vi "FPGA SECONDARY 9049.vi"() -> ()   [LabVIEW 2018]
doc: "This FPGA Main VI contains a control loop running in parallel with an RT watchdog loop.\n- The Control Loop performs control calculations on four input channels in parallel, and outputs the results to four output channels.\n- The RT Watchdog Loop checks for a periodic 'pet' from the RT Main VI to ensure communications between RT and FPGA are maintained."
uses:
  <vilib>/LabVIEW Targets/FPGA/cRIO/shared/nicrio_ModuleControls/nicrio_cRIO-9237_DataRatesRing.ctl
  <vilib>/LabVIEW Targets/FPGA/cRIO/shared/nicrio_ModuleControls/nicrio_cRIO-9237_ExcitationVoltageRing.ctl
  <vilib>/rvi/Emulation/niFpgaGetClockAttributes.vi
  <vilib>/rvi/Emulation/niFpgaSctlEmulationGetInTimedLoop.vi
  <vilib>/rvi/Emulation/niFpgaEmulationReportErrorSimple.vi
  <vilib>/rvi/eio/common/nirviEmuTemplatePropertySet_errors.vi
  <vilib>/rvi/interface/RandomDataEmulation/niFpgaRandomDataHandleErrors.vi
  <vilib>/rvi/Emulation/niFpgaProcessEmulError.vi
  <vilib>/rvi/eio/common/nirviEmuTemplateMethod_errors.vi
  <vilib>/rvi/Emulation/niFpgaCriticalErrorInLSC.vi
  <vilib>/rvi/eio/common/nirviEmuTemplatePropertyGet_noerrors.vi
  <vilib>/eio/EIOPropertyNode/EIOPropertyNode.xnode
  <vilib>/rvi/DataTransferAndStorage/Container/XNode/niFpgaContainer.xnode
  <vilib>/rvi/interface/RandomDataEmulation/nirviRandomDataFpgaReadWriteTemplate.vi
  <vilib>/eio/EIONode/EIONode.xnode
  <vilib>/eio/EIOMethodNode/EIOMethodNode.xnode
  <vilib>/rvi/eio/common/nirviEmuTemplatePropertyGet_errors.vi
  <vilib>/rvi/eio/common/nirviEmuTemplatePropertySet_noerrors.vi
  COMET  Extra Programs/FPGA Time Keeper/FPGA Timekeeper.lvlib
panel:
  out "UTC Offset Valid":bool
  out "FPGA time (ns)":u64
  out "PPS Timestamp (TAI)":u64
  out "UTC Offset":i8
  out "Antenna Status":T1(ring)
  out "offset from time reference":i32
  out "FPGA Timekeeper locked":bool
  out "FPGA Error 3":errorcluster
  out "Finished 2":bool
  out "Module Underflow 2":bool
  out "DMA FIFO Full 2":bool
  out "Different Channel Count 2":bool
  out "Actual Loop Period (ticks) 2":u32
  in  "9222 Sample Time":u32=2 caption="Sample Time 9222 [microS]"
  in  "stop":bool
  out "First Read 2":bool
  in  "Number of Channels 9222":i32=29
  out "FPGA Error 2":errorcluster
  in  "Samples per Channel":u32=1000
  in  "Finite?":bool=TRUE
  in  "Shunt Cal Enable":bool
  out "x+y 7":u8
  out "x+y 6":u8
  out "x+y 5":u8
  out "x+y 4":u8
  out "x+y 3":u8
  out "x+y":u8
  out "Preloop":i32
  out "Counter":i32
  out "appended array":fxp<+/-,24,-4>[](array[numeric])
  in  "Excitation Voltage":T2=1 items=["2.5 Volts", "3.3 Volts", "5.0 Volts", "10.0 Volts", "External Excitation"]
  out "FPGA Error":errorcluster
  out "Finished":bool
  in  "Stop":bool
  out "Module Underflow":bool
  out "DMA FIFO Full":bool
  out "Different Channel Count":bool
  out "First Read":bool
  in  "Number of Channels 9237":i32=8
  in  "Data Rate 9237":T3=1 items=["50.000 kS/s (NI 9237)"=1, "25.000 kS/s (NI 9237)"=2, "16.667 kS/s (NI 9237)"=3, "12.500 kS/s (NI 9237)"=4, "10.000 kS/s (NI 9237)"=5, "8.333 kS/s (NI 9237)"=6, "7.143 kS/s (NI 9237)"=7, "6.250 kS/s (NI 9237)"=8, "5.556 kS/s (NI 9237)"=9, "5.000 kS/s (NI 9237)"=10, "4.545 kS/s (NI 9237)"=11, "4.167 kS/s (NI 9237)"=12, "3.846 kS/s (NI 9237)"=13, "3.571 kS/s (NI 9237)"=14, "3.333 kS/s (NI 9237)"=15, "3.125 kS/s (NI 9237)"=16, "2.941 kS/s (NI 9237)"=17, "2.778 kS/s (NI 9237)"=18, "2.632 kS/s (NI 9237)"=19, "2.500 kS/s (NI 9237)"=20, "2.381 kS/s (NI 9237)"=21, "2.273 kS/s (NI 9237)"=22, "2.174 kS/s (NI 9237)"=23, "2.083 kS/s (NI 9237)"=24, "2.000 kS/s (NI 9237)"=25, "1.923 kS/s (NI 9237)"=26, "1.852 kS/s (NI 9237)"=27, "1.786 kS/s (NI 9237)"=28, "1.724 kS/s (NI 9237)"=29, "1.667 kS/s (NI 9237)"=30, "1.613 kS/s (NI 9237)"=31]
  out "Watchdog Timed Out? 2":bool=TRUE
  out "Watchdog Timed Out?":bool=TRUE
  in  "Enable Watchdog":bool
  in  "Pet Watchdog":bool
  in  "Watchdog Timeout Period (ticks)":u64=40000000 format="%.0p"
  out "Time Since Last Pet":u64
  # "Watchdog Settings"
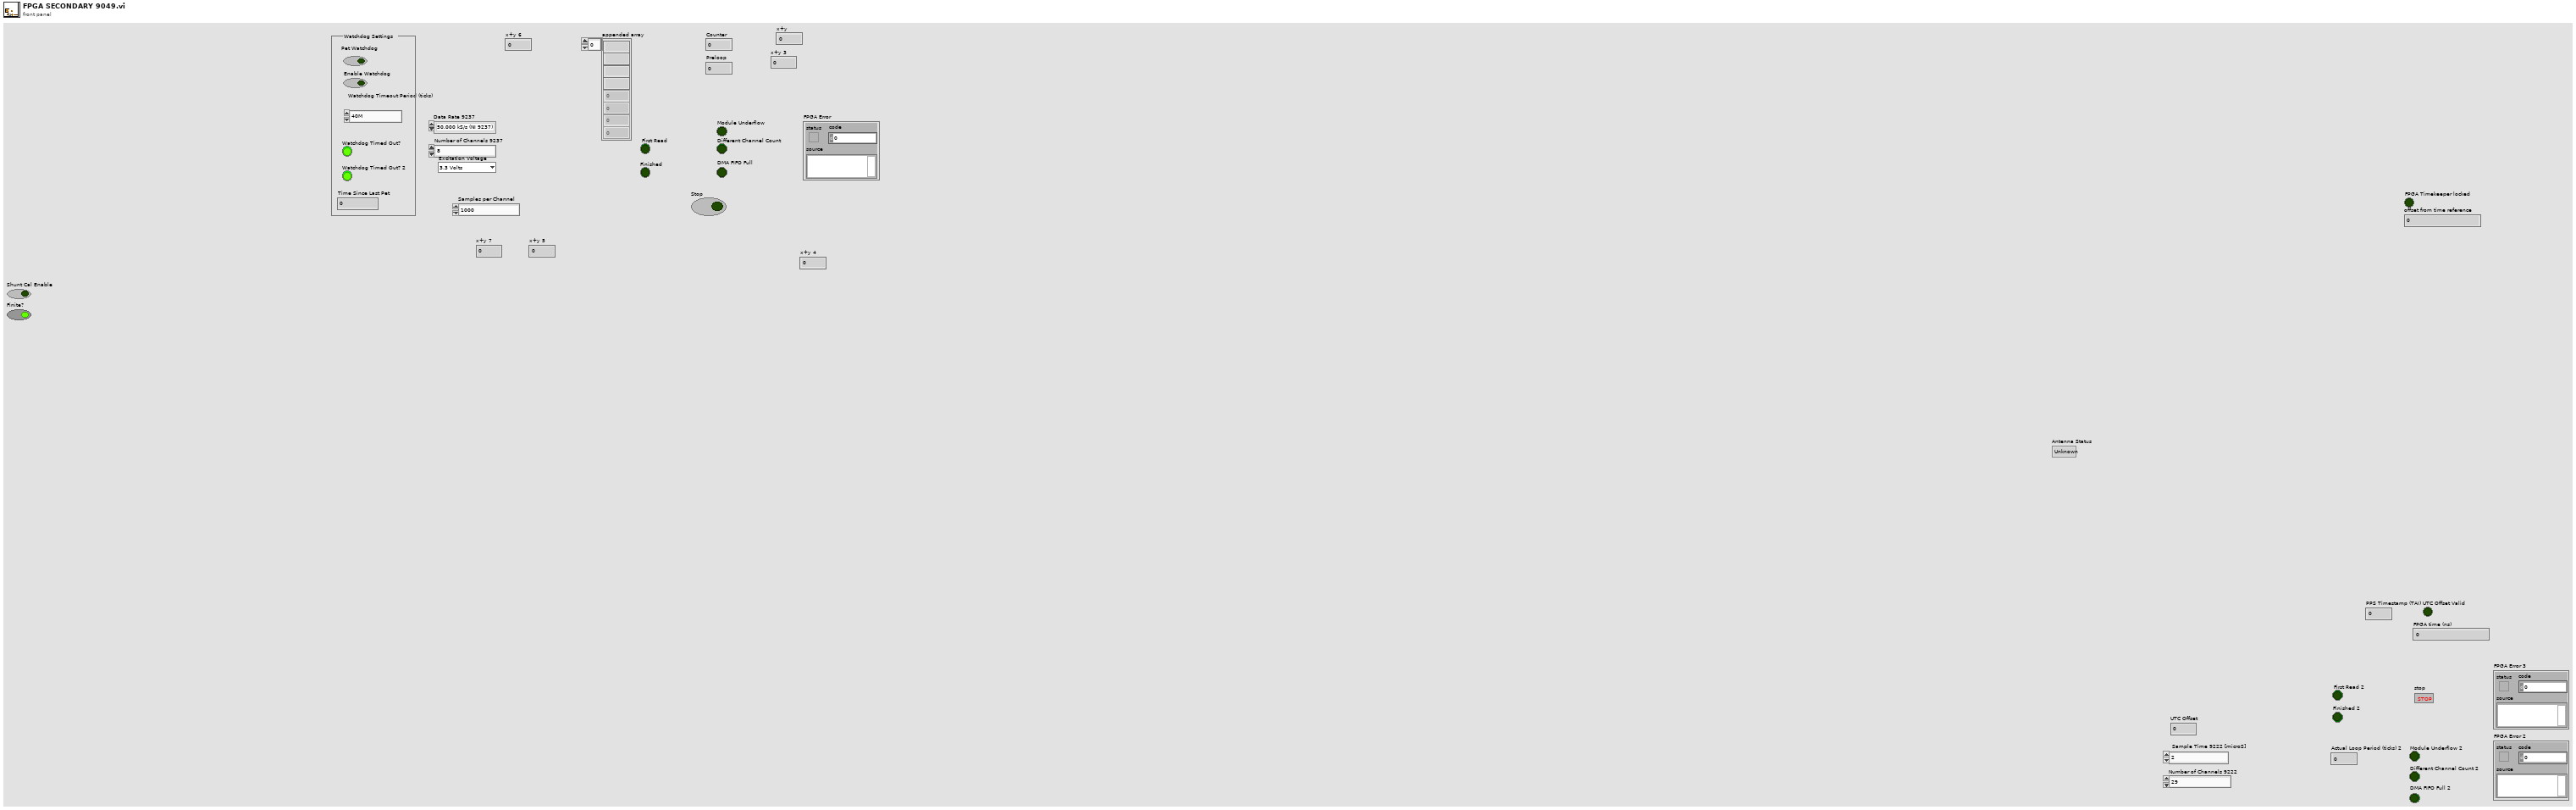
[diagram p1: front panel]
types:
  T1 = enum8{"Unknown", "Normal", "Absent", "Overcurrent"}
  T2 = typedef "nicrio_cRIO-9237_ExcitationVoltageRing.ctl" = u8
  T3 = typedef "nicrio_cRIO-9237_DataRatesRing.ctl" = u8
  T4 = enum8{"Initializing", "Normal", "Unable to get fix"}
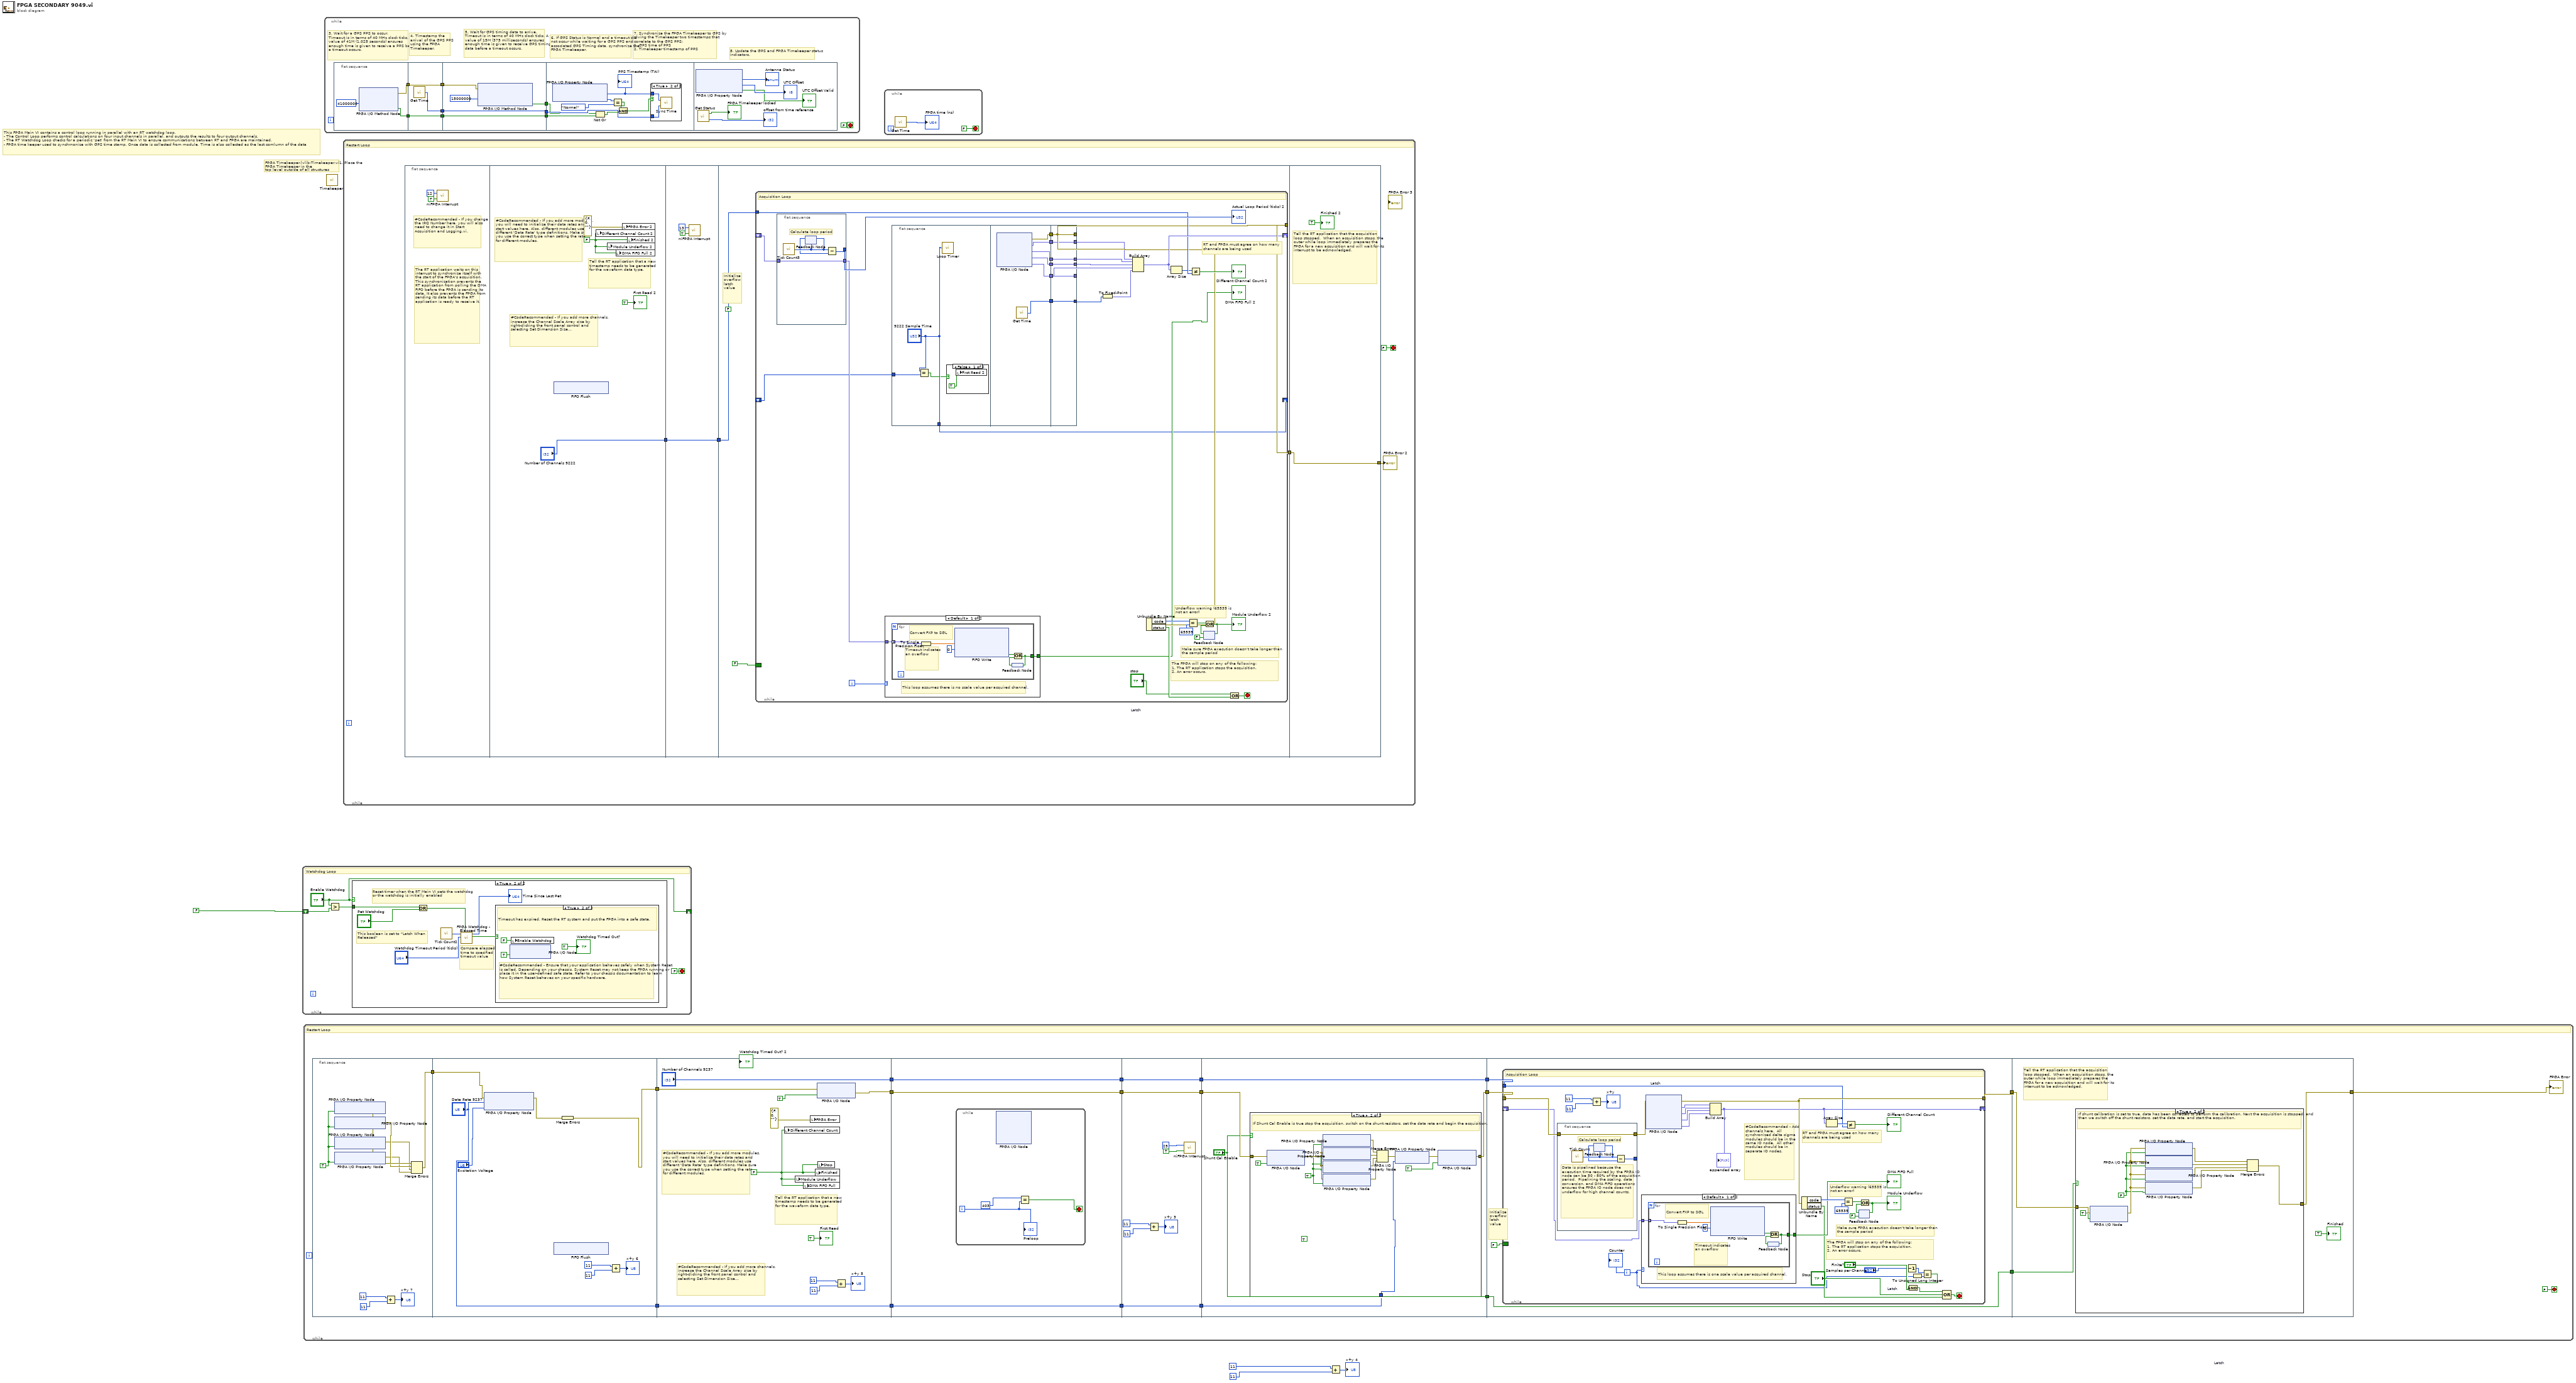
[diagram p0: block diagram]
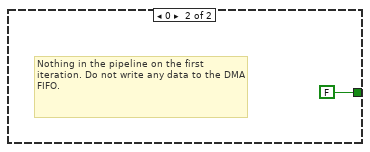
[diagram p4: hidden frame]
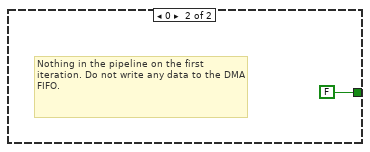
[diagram p6: hidden frame]
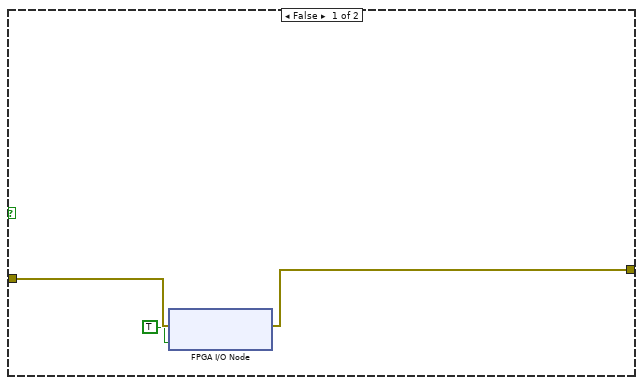
[diagram p7: hidden frame]
diagram:
  # "FPGA Timekeeper.lvlib:Timekeeper.vi1. Place the FPGA Timekeeper in the\ntop level outside of all structures"
  # "This FPGA Main VI contains a control loop running in parallel with an RT watchdog loop.\n- The Control Loop performs control calculations on four input channels in parallel, and outputs the results to four output channels.\n- The RT Watchdog Loop checks for a periodic 'pet' from the RT Main VI to ensure communications between RT and FPGA are maintained.\n- FPGA time keeper used to synchrnonize with GPS time stamp. Once data is collected from module, Time is also collected as the last comlumn of the data"
  n1 = while "RT Watchdog Loop" {
    shift-right: ["Enable Watchdog"] -> _
    shift-left: FALSE ("Enable RT Watchdog") -> [w8]
    stop <- FALSE stop-if-true
    # "Watchdog Loop"
    n2 = Greater?(x="Enable Watchdog", y=w8) -> (0:w5:bool)
    n3 = case shown="True" "Enable Watchdog" {
      tunnel: w5 -> [_ w11]
      frame False {
        # "This loop has to be explicitly enabled from the RT Main VI.  This reduces the possiblity of an endless reboot cycle."
      }
      frame True {
        # "This boolean is set to \"Latch When Released\""
        # "Compare elapsed time to specified timeout value"
        # "Reset timer when the RT Main VI pets the watchdog or the watchdog is initially enabled"
        n4 = Or(x=w11, y="Pet Watchdog") -> (x .or. y?=w10:bool)
        n5 = call "Tick Count2"() -> ("Tick Count(Ticks)"=w14:u32)
        n6 = call "FPGA Watchdog - Elapsed Time.vi"("Reset"=w10, "Timeout Period"="Watchdog Timeout Period (ticks)", "Current Time"=w14) -> ("Timeout"=w9:bool, "Elapsed Time"=→"Time Since Last Pet":u64)  [unwired: 7 in]
        n7 = case shown="True" w9 {
          frame False {
            # "Timeout has not expired."
          }
          frame True {
            # "#CodeRecommended - Ensure that your application behaves safely when System Reset is called. Depending on your chassis, System Reset may not keep the FPGA running or place it in the user-defined safe state. Refer to your chassis documentation to learn how System Reset behaves on your specific hardware."
            # "Timeout has expired. Reset the RT system and put the FPGA into a safe state."
            n8 = xnode "FPGA I/O Node"("System Reset"=TRUE ("RT Reset on Watchdog Failure?")) -> ()  [unwired: 1 in, 1 out]
            n9 = local write "Enable Watchdog"(FALSE ("Enable RT Watchdog")) -> ()
            "Watchdog Timed Out?" <- TRUE ("Watchdog Timed Out?")
          }
        }
      }
    }
  }
  n10 = while {
    stop <- FALSE stop-if-true
    # "Restart Loop"
    n11 = flat-sequence {
      tunnel: [w39] -> w23
      tunnel: [w50] -> w30
      tunnel: w23 -> [w48]
      tunnel: ["Data Rate 9237"] -> w22
      tunnel: [w62] -> w34
      tunnel: ["Number of Channels 9237"] -> w33
      tunnel: w30 -> [w61]
      tunnel: w22 -> [w55]
      tunnel: [w55] -> w21
      tunnel: w34 -> [w68]
      tunnel: [w68] -> w32
      tunnel: w33 -> [w67]
      tunnel: [w67] -> w31
      tunnel: w21 -> [w66]
      tunnel: [w66] -> w20
      tunnel: w32 -> [w79]
      tunnel: [w79] -> w29
      tunnel: w31 -> [w78]
      tunnel: [w78] -> w28
      tunnel: w20 -> [w72]
      tunnel: [w72] -> w19
      tunnel: w29 -> [w83]
      tunnel: w28 -> [w84]
      tunnel: [w84] -> w27
      tunnel: [w82] -> w26
      tunnel: ["Shunt Cal Enable"] -> w25
      tunnel: w19 -> [w80]
      tunnel: w27 -> [w103]
      tunnel: [w101] -> w36
      tunnel: w26 -> [w102]
      tunnel: w25 -> [w99]
      tunnel: [w99] -> w24
      tunnel: w36 -> [w151]
      tunnel: [w150] -> w35
      tunnel: w24 -> [w149]
      frame #0 {
        w38 = TRUE
        n12 = xnode "FPGA I/O Property Node"("Half-Bridge Enable"=w38) -> ("error out"=w43:errorcluster)  [unwired: 2 in, 1 out]
        n13 = xnode "FPGA I/O Property Node"("Half-Bridge Enable"=w38) -> ("error out"=w42:errorcluster)  [unwired: 2 in, 1 out]
        n14 = xnode "FPGA I/O Property Node"("Half-Bridge Enable"=w38) -> ("error out"=w41:errorcluster)  [unwired: 2 in, 1 out]
        n15 = xnode "FPGA I/O Property Node"("Half-Bridge Enable"=w38) -> ("error out"=w40:errorcluster)  [unwired: 2 in, 1 out]
        n16 = Add(x=u8 11 ("IRQ Number (0)"), y=u8 11 ("IRQ Number (0)")) -> (x+y=→"x+y 7":u8)
        n17 = Merge Errors(w43, w42, w41, w40) -> (w39:errorcluster)
      }
      frame #1 {
        n18 = xnode "FPGA I/O Property Node"("error in"=w48, "Data Rate"="Data Rate 9237", "Excitation Voltage"="Excitation Voltage") -> ("error out"=w51:errorcluster)  [unwired: 1 in, 1 out]
        n19 = xnode ("FIFO Flush")() -> ()  [unwired: 1 in, 1 out]
        n20 = Merge Errors(w51) -> (w50:errorcluster)
        n21 = Add(x=u8 11 ("IRQ Number (0)"), y=u8 11 ("IRQ Number (0)")) -> (x+y=→"x+y 6":u8)
      }
      frame #2 {
        w60 = FALSE ("Module Underflow")
        # "Tell the RT application that a new timestamp needs to be generated for the waveform data type."
        # "#CodeRecommended - If you add more channels, increase the Channel Scale Array size by right-clicking the front panel control and selecting Set Dimension Size..."
        # "#CodeRecommended - If you add more modules, you will need to initialize their data rates and start values here. Also, different modules use different 'Data Rate' type definitions. Make sure you use the correct type when setting the rate for different modules."
        n22 = local write "Different Channel Count"(w60) -> ()
        n23 = local write "Module Underflow"(w60) -> ()
        n24 = local write "DMA FIFO Full"(w60) -> ()
        n25 = local write "FPGA Error"(errorcluster {"status"=FALSE, "code"=0, "source"=""} ("FPGA Error")) -> ()
        n26 = local write "Finished"(w60) -> ()
        n27 = xnode "FPGA I/O Node"("error in"=w61, "Mod1/Start"=TRUE) -> ("error out"=w62:errorcluster)  [unwired: 1 in, 1 out]
        n28 = local write "Stop"(w60) -> ()
        n29 = Add(x=u8 11 ("IRQ Number (0)"), y=u8 11 ("IRQ Number (0)")) -> (x+y=→"x+y 5":u8)
        "First Read" <- TRUE ("First Read")
      }
      frame #3 {
        n30 = while {
          i -> [w69]
          stop <- w71 stop-if-true
          n31 = xnode "FPGA I/O Node"() -> ()  [unwired: 4 in, 8 out]
          n32 = Equal?(x=i16 403, y=w69) -> (x = y?=w71:bool)
          "Preloop" <- w69
        }
      }
      frame #4 {
        n33 = Add(x=u8 11 ("IRQ Number (0)"), y=u8 11 ("IRQ Number (0)")) -> (x+y=→"x+y 3":u8)
        n34 = call <vilib>:"niFPGA Interrupt.vi"("Wait Until Cleared (F)"=TRUE, "IRQ Number (0)"=u8 25) -> ()  [unwired: 1 in]
      }
      frame #5 {
        n35 = case shown="True" "Shunt Cal Enable" {
          tunnel: w83 -> [w85 w95]
          tunnel: [w85 w94] -> w82
          tunnel: w80 -> [_ w86]
          frame False {
          }
          frame True {
            (unwired) TRUE ("Shunt Cal Enable")
            w87 = TRUE ("Shunt Cal Enable")
            # "If Shunt Cal Enable is true stop the acquisition, switch on the shunt resistors, set the data rate and begin the acquisition."
            n36 = xnode "FPGA I/O Node"("error in"=w95, "Mod1/Stop"=TRUE) -> ("error out"=w91:errorcluster)  [unwired: 1 in, 1 out]
            n37 = xnode "FPGA I/O Property Node"("error in"=w91, "Shunt Cal Enable"=w87) -> ("error out"=w98:errorcluster)  [unwired: 1 in, 1 out]
            n38 = xnode "FPGA I/O Property Node"("error in"=w91, "Shunt Cal Enable"=w87) -> ("error out"=w93:errorcluster)  [unwired: 1 in, 1 out]
            n39 = xnode "FPGA I/O Property Node"("error in"=w91, "Shunt Cal Enable"=w87) -> ("error out"=w97:errorcluster)  [unwired: 1 in, 1 out]
            n40 = xnode "FPGA I/O Property Node"("error in"=w91, "Shunt Cal Enable"=w87) -> ("error out"=w96:errorcluster)  [unwired: 1 in, 1 out]
            n41 = Merge Errors(w98, w93, w97, w96) -> (w92:errorcluster)
            n42 = xnode "FPGA I/O Property Node"("error in"=w92, "Data Rate"=w86) -> ("error out"=w90:errorcluster)  [unwired: 1 in, 1 out]
            n43 = xnode "FPGA I/O Node"("error in"=w90, "Mod1/Start"=TRUE) -> ("error out"=w94:errorcluster)  [unwired: 1 in, 1 out]
          }
        }
      }
      frame #6 {
        # "Initialize overflow latch value"
        n44 = while {
          tunnel: w102 -> [w127]
          tunnel: [w132] -> w101
          shift-right: [w121] -> _
          shift-left: _ -> [w114]
          tunnel: w103 -> [w129]
          border: FALSE ("Overflow\nLatch") -> [_]
          i -> [w106]
          stop <- w135 stop-if-true
          # "Underflow warning (65539 is not an error)"
          # "The FPGA will stop on any of the following:\n1. The RT application stops the acquisition.\n2. An error occurs."
          # "#CodeRecommended - Add channels here.  All synchronized delta sigma modules should be in the same IO node.  All other modules should be in separate IO nodes."
          # "RT and FPGA must agree on how many channels are being used"
          # "Make sure FPGA execution doesn't take longer than the sample period"
          # "Acquisition Loop"
          n45 = flat-sequence {
            tunnel: [w148] -> w126
            tunnel: w127 -> [w148]
            tunnel: [w145] -> _
            frame #0 {
              # "Data is pipelined because the execution time required by the FPGA IO node can be 50 - 80% of the acquisition period.  Pipelining the scaling, data conversion, and DMA FIFO operations ensures the FPGA IO node does not underflow for high channel counts."
              # "Calculate loop period"
              n46 = call "Tick Count"() -> ("Tick Count(Ticks)"=w147:u32)
              n47 = feedback-in #1(w147) -> ()
              n48 = feedback #1(w147) -> (w146:u32)
              n49 = Subtract(x=w147, y=w146) -> (x-y=w145:u32)
            }
          }
          n50 = Add(x=u8 11 ("IRQ Number (0)"), y=u8 11 ("IRQ Number (0)")) -> (x+y=→"x+y":u8)
          n51 = case shown="Default" w106 {
            tunnel: [w137 FALSE] -> w131
            tunnel: w114 -> [w136 _]
            frame Default {
              # "This loop assumes there is one scale value per acquired channel."
              n52 = for {
                tunnel: [w141] -> w137
                tunnel: w136 -> [w138] mode=indexing
                # "Timeout indicates an overflow"
                # "Convert FXP to SGL"
                n53 = To Single Precision Float(number=w138) -> (single precision float=w139:sgl)
                n54 = xnode ("FIFO Write")("Element"=w139, "Timeout"=0) -> ("Timed Out?"=w143:bool)  [unwired: 1 in, 1 out]
                n55 = feedback #2 "Latch"() -> (w142:bool)
                n56 = Or(x=w143, y=w142) -> (x .or. y?=w141:bool)
                n57 = feedback-in #2(w141) -> ()
              }
            }
            frame 0 {
              # "Nothing in the pipeline on the first iteration. Do not write any data to the DMA FIFO."
            }
          }
          "DMA FIFO Full" <- w131
          n58 = xnode "FPGA I/O Node"("error in"=w126) -> ("error out"=w132:errorcluster, "Mod1/AI0"=w125:fxp<+/-,24,-4>, "Mod1/AI1"=w122:fxp<+/-,24,-4>, "Mod1/AI2"=w124:fxp<+/-,24,-4>, "Mod1/AI3"=w123:fxp<+/-,24,-4>)  [unwired: 4 in, 4 out]
          n59 = Build Array(w125, w122, w124, w123) -> (w121:fxp<+/-,24,-4>[])
          "appended array" <- w121
          n60 = Unbundle By Name(w132) -> ("code"=w133:i32, "status"=w116:bool)
          n61 = Array Size(array=w121) -> (size(s)=w130:i32)
          n62 = Equal?(x=w133, y=65539) -> (x = y?=w118:bool)
          n63 = Not Equal?(x=w130, y=w129) -> (x != y?=→"Different Channel Count":bool)
          n64 = feedback #3 "Latch"(FALSE) -> (w120:bool)
          n65 = Or(x=w118, y=w120) -> (x .or. y?=w117:bool)
          "Module Underflow" <- w117
          n66 = feedback-in #3(w117) -> ()
          n67 = Decrement(x="Samples per Channel") -> (x-1=w109:u32)
          n68 = To Unsigned Long Integer(number=w106) -> (unsigned 32bit integer=w110:u32)
          n69 = Equal?(x=w109, y=w110) -> (x = y?=w105:bool)
          n70 = And(x=w105, y="Finite?") -> (x .and. y?=w104:bool)
          n71 = Compound Arithmetic op=OR(w104, "Stop", w116) -> (w135:bool)
          "Counter" <- w106
        }
      }
      frame #7 {
        # "Tell the RT application that the acquisition loop stopped.  When an acquisition stops, the outer while loop immediately prepares the FPGA for a new acquisition and will wait for its interrupt to be acknowledged."
        n72 = case shown="True" w149 {
          tunnel: w151 -> [w155 w160]
          tunnel: [w154 w159] -> w150
          frame False {
            n73 = xnode "FPGA I/O Node"("error in"=w155, "Mod1/Stop"=TRUE) -> ("error out"=w154:errorcluster)  [unwired: 1 in, 1 out]
          }
          frame True {
            w156 = FALSE ("Shunt Cal Enable")
            # "If shunt calibration is set to true, data has been collected to perform the calibration. Next the acquisition is stopped, and then we switch off the shunt resistors, set the data rate, and start the acquisition."
            n74 = xnode "FPGA I/O Node"("error in"=w160, "Mod1/Stop"=TRUE) -> ("error out"=w157:errorcluster)  [unwired: 1 in, 1 out]
            n75 = xnode "FPGA I/O Property Node"("error in"=w157, "Shunt Cal Enable"=w156) -> ("error out"=w164:errorcluster)  [unwired: 1 in, 1 out]
            n76 = xnode "FPGA I/O Property Node"("error in"=w157, "Shunt Cal Enable"=w156) -> ("error out"=w163:errorcluster)  [unwired: 1 in, 1 out]
            n77 = xnode "FPGA I/O Property Node"("error in"=w157, "Shunt Cal Enable"=w156) -> ("error out"=w162:errorcluster)  [unwired: 1 in, 1 out]
            n78 = xnode "FPGA I/O Property Node"("error in"=w157, "Shunt Cal Enable"=w156) -> ("error out"=w161:errorcluster)  [unwired: 1 in, 1 out]
            n79 = Merge Errors(w164, w163, w162, w161) -> (w159:errorcluster)
          }
        }
        "Finished" <- TRUE ("Finished")
      }
    }
    "FPGA Error" <- w35
  }
  n80 = while {
    stop <- FALSE stop-if-true
    # "3. Wait for a GPS PPS to occur.\nTimeout is in terms of 40 MHz clock ticks. A value of 41M (1.025 seconds) ensures enough time is given to receive a PPS before a timeout occurs."
    # "4. Timestamp the arrival of the GPS PPS using the FPGA Timekeeper."
    # "6. If GPS Status is Normal and a timeout did not occur while waiting for a GPS PPS and associated GPS Timing data, synchronize the FPGA Timekeeper."
    # "7. Synchronize the FPGA Timekeeper to GPS by giving the Timekeeper two timestamps that correlate to the GPS PPS:\n1. GPS time of PPS\n2. Timekeeper timestamp of PPS"
    # "5. Wait for GPS timing data to arrive.\nTimeout is in terms of 40 MHz clock ticks. A value of 15M (375 milliseconds) ensures enough time is given to receive GPS timing data before a timeout occurs."
    # "8. Update the GPS and FPGA Timekeeper status indicators."
    n81 = flat-sequence {
      tunnel: [w175] -> w171
      tunnel: [w174] -> w166
      tunnel: [w179] -> w172
      tunnel: w171 -> [w179]
      tunnel: [w178] -> w169
      tunnel: w166 -> [w177]
      tunnel: [w177] -> w165
      tunnel: [w183] -> w173
      tunnel: w172 -> [w183]
      tunnel: [w182] -> w170
      tunnel: w169 -> [w181]
      tunnel: [w181] -> w168
      tunnel: w165 -> [w180]
      tunnel: w168 -> [w192]
      tunnel: w170 -> [w186]
      tunnel: w173 -> [w187]
      frame #0 {
        n82 = xnode "FPGA I/O Method Node"("Timeout"=41000000) -> ("error out"=w174:errorcluster, "Timed Out"=w175:bool)  [unwired: 2 in, 1 out]
      }
      frame #1 {
        n83 = call "Get Time.vi"() -> ("time (ns)"=w178:u64)
      }
      frame #2 {
        n84 = xnode "FPGA I/O Method Node"("error in"=w180, "Timeout"=15000000) -> ("Timed Out"=w182:bool)  [unwired: 1 in, 2 out]
      }
      frame #3 {
        n85 = xnode "FPGA I/O Property Node"() -> ("PPS Timestamp (TAI)"=w191:u64, "GPS Status"=w190:T4)  [unwired: 1 in, 1 out]
        "PPS Timestamp (TAI)" <- w191
        n86 = Not Or(1:w187, 2:w186) -> (0:w185:bool)
        n87 = Equal?(x=w190, y=T4."Normal" ("GPS Status")) -> (x = y?=w188:bool)
        n88 = And(x=w188, y=w185) -> (x .and. y?=w193:bool)
        n89 = case shown="True" w193 {
          tunnel: w192 -> [_ w195]
          tunnel: w191 -> [_ w194]
          frame False {
          }
          frame True {
            n90 = call "Sync Time.vi"("FPGA Timekeeper time (ns)"=w195, "time reference time (ns)"=w194) -> ()
          }
        }
      }
      frame #4 {
        n91 = xnode "FPGA I/O Property Node"() -> ("Antenna Status"=→"Antenna Status":T1, "UTC Offset"=→"UTC Offset":i8, "UTC Offset Valid"=→"UTC Offset Valid":bool)  [unwired: 1 in, 1 out]
        n92 = call "Get Status.vi"() -> ("FPGA Timekeeper locked"=→"FPGA Timekeeper locked":bool, "offset from time reference"=→"offset from time reference":i32)
      }
    }
  }
  n93 = call "Timekeeper.vi"() -> ()  [unwired: 12 in]
  n94 = while {
    stop <- FALSE stop-if-true
    # "Restart Loop"
    n95 = flat-sequence {
      tunnel: ["Number of Channels 9222"] -> w202
      tunnel: w202 -> [w214]
      tunnel: [w214] -> w201
      tunnel: w201 -> [w217]
      tunnel: [w215] -> w204
      tunnel: w204 -> [w280]
      tunnel: [w280] -> w203
      frame #0 {
        # "#CodeRecommended - If you change the IRQ Number here, you will also need to change it in Start Acquisition and Logging.vi."
        # "The RT application waits on this interrupt to synchronize itself with the start of the FPGA's acquisition.  This synchronization prevents the RT application from polling the DMA FIFO before the FPGA is sending its data. It also prevents the FPGA from sending its data before the RT application is ready to receive it."
        n96 = call <vilib>:"niFPGA Interrupt.vi"("Wait Until Cleared (F)"=TRUE, "IRQ Number (0)"=u8 12) -> ()  [unwired: 1 in]
      }
      frame #1 {
        w210 = FALSE ("Module Underflow")
        # "Tell the RT application that a new timestamp needs to be generated for the waveform data type."
        # "#CodeRecommended - If you add more channels, increase the Channel Scale Array size by right-clicking the front panel control and selecting Set Dimension Size..."
        # "#CodeRecommended - If you add more modules, you will need to initialize their data rates and start values here. Also, different modules use different 'Data Rate' type definitions. Make sure you use the correct type when setting the rate for different modules."
        n97 = xnode ("FIFO Flush")() -> ()  [unwired: 1 in, 1 out]
        n98 = local write "Different Channel Count 2"(w210) -> ()
        n99 = local write "Module Underflow 2"(w210) -> ()
        n100 = local write "DMA FIFO Full 2"(w210) -> ()
        n101 = local write "FPGA Error 2"(errorcluster {"status"=FALSE, "code"=0, "source"=""} ("FPGA Error")) -> ()
        n102 = local write "Finished 2"(w210) -> ()
        "First Read 2" <- TRUE ("First Read")
      }
      frame #2 {
        n103 = call <vilib>:"niFPGA Interrupt.vi"("Wait Until Cleared (F)"=TRUE, "IRQ Number (0)"=u8 13) -> ()  [unwired: 1 in]
      }
      frame #3 {
        (unwired) FALSE ("Overflow\nLatch")
        # "Initialize overflow latch value"
        n104 = while {
          tunnel: [w236] -> w215
          shift-right: [w245] -> _
          shift-left: _ -> [w237]
          tunnel: w217 -> [w239]
          border: FALSE ("Overflow\nLatch") -> [_]
          shift-right: [w227] -> _
          shift-left: _ -> [w226]
          i -> [w230]
          stop <- w250 stop-if-true
          # "Underflow warning (65539 is not an error)"
          # "The FPGA will stop on any of the following:\n1. The RT application stops the acquisition.\n2. An error occurs."
          # "RT and FPGA must agree on how many channels are being used"
          # "Make sure FPGA execution doesn't take longer than the sample period"
          # "Acquisition Loop"
          n105 = flat-sequence {
            tunnel: [w277] -> w246
            tunnel: [w276] -> w238
            tunnel: w237 -> [w276]
            frame #0 {
              # "Calculate loop period"
              n106 = call "Tick Count3"() -> ("Tick Count(Ticks)"=w279:u32)
              n107 = feedback-in #4(w279) -> ()
              n108 = feedback #4(w279) -> (w278:u32)
              n109 = Subtract(x=w279, y=w278) -> (x-y=w277:u32)
            }
          }
          n110 = case shown="Default" w230 {
            tunnel: [w268 FALSE] -> w229
            tunnel: w238 -> [w267 _]
            frame Default {
              # "This loop assumes there is no scale value per acquired channel."
              n111 = for {
                tunnel: [w272] -> w268
                tunnel: w267 -> [w269] mode=indexing
                # "Timeout indicates an overflow"
                # "Convert FXP to SGL"
                n112 = To Single Precision Float(number=w269) -> (single precision float=w270:sgl)
                n113 = xnode ("FIFO Write")("Element"=w270, "Timeout"=0) -> ("Timed Out?"=w274:bool)  [unwired: 1 in, 1 out]
                n114 = feedback #5 "Latch"() -> (w273:bool)
                n115 = Or(x=w274, y=w273) -> (x .or. y?=w272:bool)
                n116 = feedback-in #5(w272) -> ()
              }
            }
            frame 0 {
              # "Nothing in the pipeline on the first iteration. Do not write any data to the DMA FIFO."
            }
          }
          "DMA FIFO Full 2" <- w229
          n117 = flat-sequence {
            tunnel: ["9222 Sample Time"] -> w227
            tunnel: w226 -> [w253]
            tunnel: [w260] -> w225
            tunnel: [w259] -> w224
            tunnel: [w258] -> w223
            tunnel: [w257] -> w222
            tunnel: [w256] -> w221
            tunnel: [w255] -> w220
            tunnel: [w262] -> w232
            tunnel: [w263] -> w233
            tunnel: [w264] -> w234
            tunnel: [w265] -> w235
            tunnel: [w266] -> w236
            tunnel: w225 -> [w266]
            tunnel: w224 -> [w265]
            tunnel: w223 -> [w264]
            tunnel: w222 -> [w263]
            tunnel: w221 -> [w262]
            tunnel: w220 -> [w261]
            tunnel: [w261] -> w219
            frame #0 {
              n118 = Equal?(x="9222 Sample Time", y=w253) -> (x = y?=w251:bool)
              n119 = call "Loop Timer"("Count(uSec)"="9222 Sample Time") -> ()  [unwired: 1 out]
              n120 = case shown="False" w251 {
                frame False {
                  n121 = local write "First Read 2"(TRUE ("First Read")) -> ()
                }
                frame True {
                }
              }
            }
            frame #1 {
              n122 = xnode "FPGA I/O Node"() -> ("error out"=w260:errorcluster, "Mod2/AI0"=w259:fxp<+/-,24,5>, "Mod2/AI1"=w258:fxp<+/-,24,5>, "Mod2/AI2"=w257:fxp<+/-,24,5>, "Mod2/AI3"=w256:fxp<+/-,24,5>)  [unwired: 5 in, 4 out]
              n123 = call "Get Time.vi"() -> ("time (ns)"=w255:u64)
            }
            frame #2 {
            }
          }
          n124 = To Fixed-Point(number=w219) -> (fixed-point=w218:fxp<+,64,64>)  [unwired: 1 in]
          n125 = Build Array(w235, w234, w233, w232, w218) -> (w245:fxp<+/-,64,65>[])
          n126 = Unbundle By Name(w236) -> ("code"=w248:i32, "status"=w240:bool)
          n127 = Array Size(array=w245) -> (size(s)=w228:i32)
          n128 = Equal?(x=w248, y=65539) -> (x = y?=w242:bool)
          n129 = Not Equal?(x=w228, y=w239) -> (x != y?=→"Different Channel Count 2":bool)
          n130 = feedback #6 "Latch"(FALSE) -> (w244:bool)
          n131 = Or(x=w242, y=w244) -> (x .or. y?=w241:bool)
          "Module Underflow 2" <- w241
          n132 = feedback-in #6(w241) -> ()
          n133 = Compound Arithmetic op=OR("stop", w240) -> (w250:bool)
          "Actual Loop Period (ticks) 2" <- w246
        }
      }
      frame #4 {
        # "Tell the RT application that the acquisition loop stopped.  When an acquisition stops, the outer while loop immediately prepares the FPGA for a new acquisition and will wait for its interrupt to be acknowledged."
        "Finished 2" <- TRUE ("Finished")
      }
    }
    "FPGA Error 2" <- w203
  }
  n134 = while {
    stop <- FALSE stop-if-true
    n135 = call "Get Time.vi"() -> ("time (ns)"=→"FPGA time (ns)":u64)
  }
  n136 = Add(x=u8 11 ("IRQ Number (0)"), y=u8 11 ("IRQ Number (0)")) -> (x+y=→"x+y 4":u8)
